vi "priv_AR_Core.vi"(7 "CoreRef":refnum<vi>, 8 "error in (no error)":errorcluster, 10 "Databox_sealed":refnum<class "Databox_sealed.lvclass">, 11 "AR_Matching":T1[](array[typedef])) -> (0 "error out":errorcluster)   [LabVIEW 2020, in "UI_Actor.lvlib" / "UI_Actor.lvclass"]
uses:
  UI_Actor.lvclass
  support/Databox.lvlibp/Databox_sealed/Databox_sealed.lvclass
  ctl_AR_Elmt.ctl
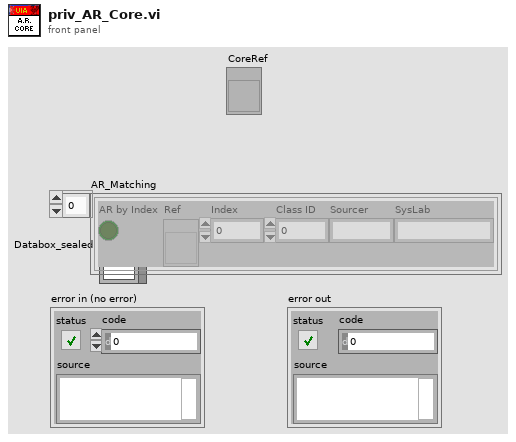
[diagram p1: front panel]
types:
  T1 = typedef "UI_Actor.lvlib/UI_Actor.lvclass/ctl_AR_Elmt.ctl" = cluster{"AR by Index":bool, "Ref":refnum<vi>, "Index":i32, "Class ID":u32, "Sourcer":string, "SysLab":string}
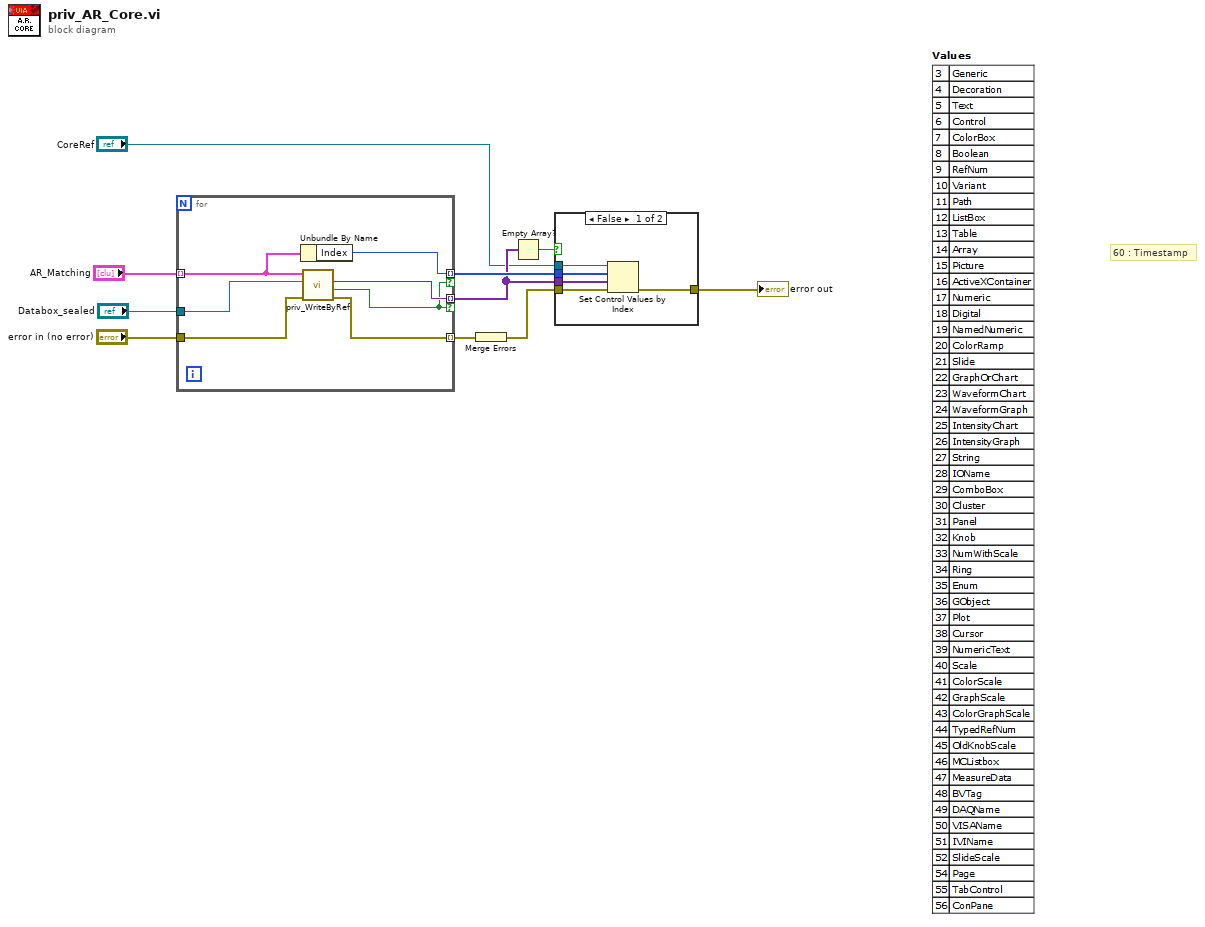
[diagram p0: block diagram]
diagram:
  # "60 : Timestamp"
  n1 = for {
    tunnel: "AR_Matching" -> [w12] mode=indexing
    tunnel: "Databox_sealed" -> [w15]
    tunnel: "error in (no error)" -> [w17]
    tunnel: [w16] -> w8 mode=indexing
    tunnel: [w11] -> w7 mode=indexing if=w13
    tunnel: [w14] -> w3 mode=indexing if=w13
    n2 = Unbundle By Name(w12) -> ("Index"=w11:i32)
    n3 = call "priv_WriteByRef.vi"("error in (no error)"=w17, "Databox_sealed"=w15, "AR_Elmt"=w12) -> ("error out"=w16:errorcluster, "Write Index"=w13:bool, "Data To Disp out"=w14:variant)  [unwired: 6 in]
  }
  n4 = Merge Errors(w8) -> (w5:errorcluster)
  n5 = Empty Array?(array=w3) -> (empty?=w2:bool)
  n6 = case shown="False" w2 {
    tunnel: w3 -> [w22 _]
    tunnel: w7 -> [w21 _]
    tunnel: "CoreRef" -> [w20 _]
    tunnel: w5 -> [w19 w23]
    tunnel: [w18 w23] -> w4
    frame False {
      n7 = Set Control Values by Index(0:w20, 1:w21, 2:w22, 3:w19) -> (11:w18:errorcluster)
    }
    frame True {
    }
  }
  "error out" <- w4
